vi "TriggerTests_1_1.vi"() -> ()   [LabVIEW 2009]
uses:
  <vilib>/Utility/NIReport.llb/NI_report.lvclass
  <vilib>/express/express signal manip/GetorSetDDTAttributes/Set DDT Attributes/Set DDT Properties.xnode
  <vilib>/express/express shared/transition.llb/Waveform Array To Dynamic.vi
  <vilib>/express/express signal manip/GetorSetDDTAttributes/Set DDT Attributes/SetT0.vi
  <vilib>/express/express shared/transition.llb/Dynamic To Waveform Array.vi
  <vilib>/express/express signal manip/GetorSetDDTAttributes/Shared VIs/XDimension Enum to String.vi
  <vilib>/express/express signal manip/GetorSetDDTAttributes/Shared VIs/XDimension.ctl
  <vilib>/express/express signal manip/GetorSetDDTAttributes/Shared VIs/GetSetShared.lvlib
panel:
  in  "Report Enable":bool=TRUE
  in  "Curve data path":path=path "D:/CTA/IntegrationBoard/tmp"
  in  "Save curves":bool=TRUE
  in  "Instrument VISA in":T1={"AWG VISA"="81160A", "Oscilloscope  VISA "="DSO80204B", "Integration Board IP"="172.16.7.43", "connection ID"=refnum, "report out"=refnum}
  out "error out":errorcluster
  out "L1 Level Above Noise":i32
  out "DT_50_L0":dbl[][](array[numeric])
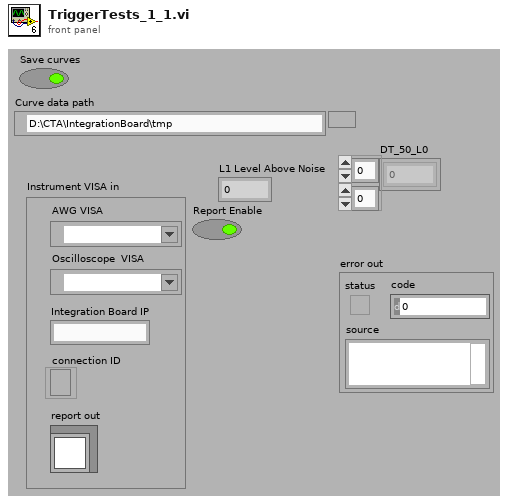
[diagram p1: front panel]
types:
  T1 = cluster{"AWG VISA":refnum<visa-resource-name>, "Oscilloscope  VISA ":refnum<visa-resource-name>, "Integration Board IP":string, "connection ID":refnum<k5>, "report out":refnum<class "NI_report.lvclass">}
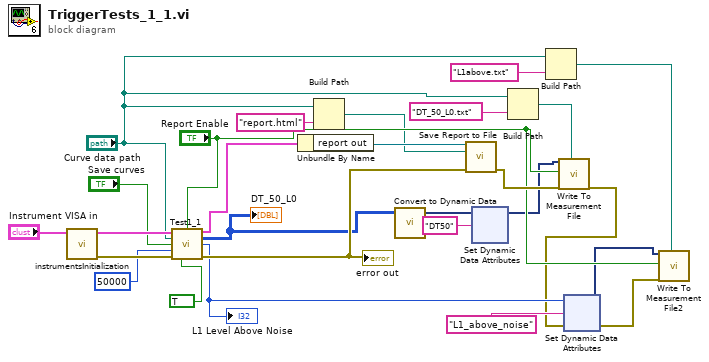
[diagram p0: block diagram]
diagram:
  n1 = call "instrumentsInitialization.vi"("Instrument VISA in"="Instrument VISA in") -> ("error out"=w27:errorcluster, "Instrument VISA out"=w24:T1)  [unwired: 9 in]
  n2 = call "Test1_1.vi"("Instrument VISA in"=w24, "Report Enable"="Report Enable", "Curve data path"="Curve data path", "Save curves"="Save curves", "Cycles Burst"=50000, "error in"=w27, "L1 version"=TRUE) -> ("Instrument VISA out"=w20:T1, "DT_50_L0"=w9:i32[][], "L1 Level Above Noise"=w6:i32, "error out"=w19:errorcluster)  [unwired: 5 in]
  "DT_50_L0" <- w9
  "L1 Level Above Noise" <- w6
  "error out" <- w19
  n3 = Unbundle By Name(w20) -> ("report out"=w21:refnum<class "NI_report.lvclass">)
  n4 = Build Path(base path="Curve data path", name or relative path="report.html") -> (appended path=w12:path)
  n5 = call "Convert to Dynamic Data"("2D Array"=w9) -> ("Dynamic Data Type"=w8:dynamicdata)  [unwired: 3 in]
  n6 = call-dynamic "Save Report to File.vi"("report in"=w21, "report file path"=w12, "error in (no error)"=w19) -> ("error out"=w18:errorcluster)  [unwired: 11 in, 1 out]
  n7 = xnode ("Set Dynamic Data Attributes")("Signals In"=w8, "Signal Name"="DT50") -> ("Signals Out"=w7:dynamicdata)  [unwired: 3 in, 1 out]
  n8 = Build Path(base path="Curve data path", name or relative path="DT_50_L0.txt" ("Comment")) -> (appended path=w13:path)
  n9 = Build Path(base path="Curve data path", name or relative path="L1above.txt") -> (appended path=w15:path)
  n10 = call "Write To Measurement File"("Signals"=w7, "Enable"="Report Enable", "error in (no error)"=w18, "Filename"=w13) -> ("error out"=w2:errorcluster)  [unwired: 13 in, 2 out]
  n11 = xnode ("Set Dynamic Data Attributes")("Signals In"=w6, "error in"=w2, "Signal Name"="L1_above_noise") -> ("Signals Out"=w5:dynamicdata, "error out"=w1:errorcluster)  [unwired: 2 in]
  n12 = call "Write To Measurement File2"("Signals"=w5, "Enable"="Report Enable", "error in (no error)"=w1, "Filename"=w15) -> ()  [unwired: 13 in, 3 out]
